vi "SetOIDNumbers.vi"(8 "error in (no error)":errorcluster, 11 "RoomAlert in":refnum<class "RoomAlert.lvclass">) -> (0 "error out":errorcluster, 3 "RoomAlert out":refnum<class "RoomAlert.lvclass">)   [LabVIEW 2018, in "SensorPlugins.lvlib" / "RoomAlert.lvclass"]
uses:
  RoomAlert.lvclass
panel:
  in  "Modle ID Array In":string[][](array[string])=[["12E", "4E"]]
  out "Modle ID ArrayOut":string[][](array[string])=[["12E", "4E"]]
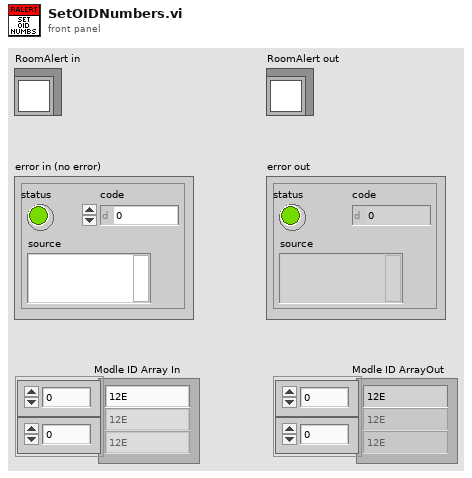
[diagram p1: front panel]
types:
  T1 = typedef "SensorPlugins.lvlib/RoomAlert.lvclass/RoomAlertControls.ctl" = cluster{"Connected?":bool, "IP Address of SNMP Device":string, "Port (161)":u16, "Community Name":string, "Measurements To Read Array":u16[], "Update LightTower?":bool, "LightTower":cluster{"Red":bool, "Amber":bool, "Green":bool, "Audio":bool}, "RoomAlert Model ID":string, "Sensor OID Numbers":string[][], "Sensor Light Tower OID Numbers":string[][]}[]
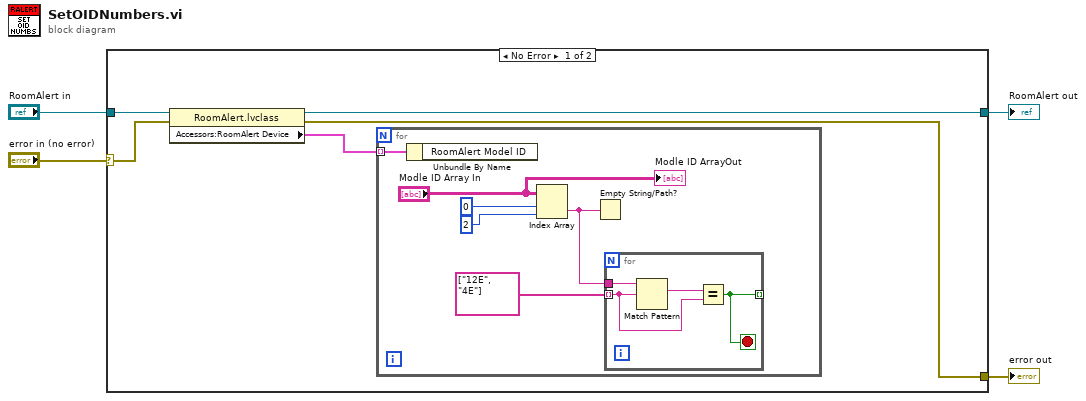
[diagram p0: block diagram]
diagram:
  n1 = case shown="No Error" "error in (no error)" {
    selector: "error in (no error)" -> [w7 w21]
    tunnel: [w5 w21] -> w3
    tunnel: [w6 w20] -> w1
    tunnel: "RoomAlert in" -> [w8 w20]
    frame No Error {
      n2 = property class="RoomAlert.lvclass"(reference=w8, error in=w7) -> (reference out=w6:refnum<class "RoomAlert.lvclass">, error out=w5:errorcluster, "Accessors:RoomAlert Device"=w9:T1)
      n3 = for {
        tunnel: w9 -> [w10] mode=indexing
        n4 = Unbundle By Name(w10) -> ()  [unwired: 1 out]
        n5 = Index Array(array="Modle ID Array In", index (row)=0, index (col)=2 ("disabled index (col)")) -> (element=w12:string)
        n6 = Empty String/Path?(string/path=w12) -> ()  [unwired: 1 out]
        n7 = for {
          tunnel: w12 -> [w19]
          tunnel: string[] ["12E", "4E"] -> [w18] mode=indexing
          tunnel: [w16] -> _ mode=indexing
          stop <- w16 stop-if-true
          n8 = Match Pattern(string=w19, regular expression=w18) -> (match substring=w17:string)  [unwired: 1 in, 3 out]
          n9 = Equal?(x=w17, y=w18) -> (x = y?=w16:bool)
        }
        "Modle ID ArrayOut" <- "Modle ID Array In"
      }
    }
    frame Error {
    }
  }
  "error out" <- w3
  "RoomAlert out" <- w1
